vi "Load Relay Map.vi"(8 "error in":errorcluster, 11 "2575 in":refnum<class "2575.lvclass">) -> (0 "error out":errorcluster, 3 "2575 out":refnum<class "2575.lvclass">)   [LabVIEW 2019, in "2575.lvlib" / "2575.lvclass"]
uses:
  Library/2575.lvclass
  C:/Users/Public/Documents/Development/builds/Instruments/SwitchMatrix.lvlibp/Library/SwitchMatrix.lvclass
  <instrlib>/niSwitch/niSwitch.llb/niSwitch Topologies.ctl
  builds/Instruments/SwitchMatrix.lvlibp/Accessors/Read Matrix Topology.vi
panel:
  in  "95 to 1":i32[](array[numeric])=[97, 93, 89, 85, 81, 77, 73, 69, 65, 61, 57, 53, 47, 44, 40, 39, 32, 28, 24, 20, 16, 11, 7, 3, 52, 56, 60, 64, 68, 72, 76, 80, 84, 87, 91, 95, 2, 6, 10, 14, 19, 23, 27, 31, 35, 38, 43, 46, 96, 92, 88, 83, 79, 75, 71, 67, 63, 59, 55, 51, 45, 42, 37, 34, 30, 26, 22, 18, 13, 9, 5, 1, 50, 54, 58, 62, 66, 70, 74, 78, 82, 86, 90, 94, 0, 4, 8, 12, 17, 21, 25, 29, 33, 36, 41]
  in  "98 to 1":i32[](array[numeric])=[97, 93, 89, 85, 81, 77, 73, 69, 65, 61, 57, 53, 47, 44, 40, 39, 32, 28, 24, 20, 16, 11, 7, 3, 52, 56, 60, 64, 68, 72, 76, 80, 84, 87, 91, 95, 2, 6, 10, 14, 19, 23, 27, 31, 35, 38, 43, 46, 96, 92, 88, 83, 79, 75, 71, 67, 63, 59, 55, 51, 45, 42, 37, 34, 30, 26, 22, 18, 13, 9, 5, 1, 50, 54, 58, 62, 66, 70, 74, 78, 82, 86, 90, 94, 0, 4, 8, 12, 17, 21, 25, 29, 33, 36, 41, 48, 49, 98]
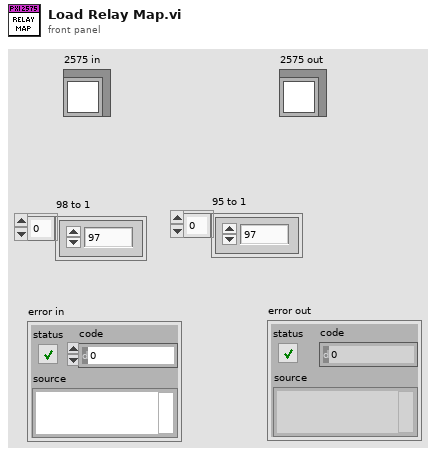
[diagram p1: front panel]
types:
  T1 = typedef "niSwitch Topologies.ctl" = string
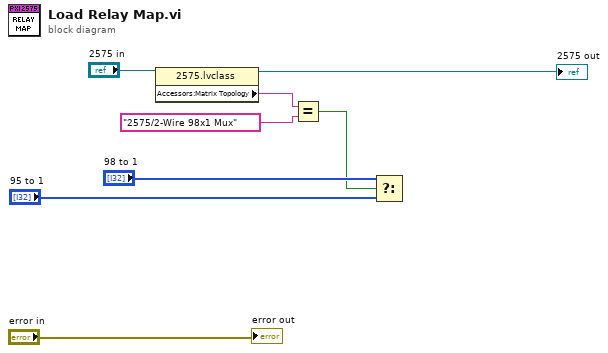
[diagram p0: block diagram]
diagram:
  n1 = property class="2575.lvclass"(reference="2575 in") -> (reference out=→"2575 out":refnum<class "2575.lvclass">, "Accessors:Matrix Topology"=w4:string)  [unwired: 1 in, 1 out]
  n2 = Equal?(x=w4, y=T1 "2575/2-Wire 98x1 Mux" ("topology name 2")) -> (x = y?=w3:bool)
  n3 = Select(t="98 to 1", s=w3, f="95 to 1") -> ()  [unwired: 1 out]
  "error out" <- "error in"
